vi "Create Relay Resources.vi"() -> (3 "state handshake":T1)   [LabVIEW 2015, in "niInstr Streaming v1 FPGA.lvlib"]
uses:
  <instrlib>/_niInstr/Streaming/v1/FPGA/niInstr Streaming v1 FPGA.lvlib
  <instrlib>/_niInstr/Streaming/v1/FPGA/Public/Stream Additive Count Register.ctl
  <vilib>/rvi/DataTransferAndStorage/Container/Common/niFpgaContainerGetUniqueNameForEmu.vi
  <vilib>/rvi/DataTransferAndStorage/Container/Common/niFpgaContainerSetEmuInfo.vi
  <vilib>/rvi/eio/common/nirviEmuReportErrorAndStop.vi
  <vilib>/rvi/LocalResourceManager/LocalResourceManager.xnode
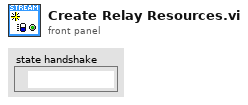
[diagram p1: front panel]
types:
  T1 = typedef "niInstr Streaming v1 FPGA.lvlib/Stream Additive Count Register.ctl" = refnum<k21>
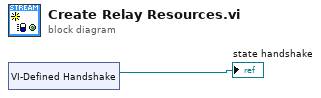
[diagram p0: block diagram]
diagram:
  n1 = xnode "VI-Defined Handshake"() -> ("Handshake Out"=→"state handshake":refnum<k21>)
